vi "main.vi"() -> ()   [LabVIEW 2021]
uses:
  Global Config.ctl
  ini Entry.ctl
  VIPM.ctl
  <userlib>/_MGI/Application Control/MGI Gray if/MGI Gray if False.vi
  <vilib>/addons/_JKI.lib/Serialization/JSON/JKI JSON Serialization.lvlib
panel:
  out "Status":string
  out "Progress Bar":dbl(slide) scale=0.0..10.0
  in  "Start":bool
  in  "LV Install Folder":path caption="LabVIEW Installation Folder (eg: C:\\Program Files (x86)\\National Instruments\\LabVIEW 2021)"
  # "LV-Custom-Settings"
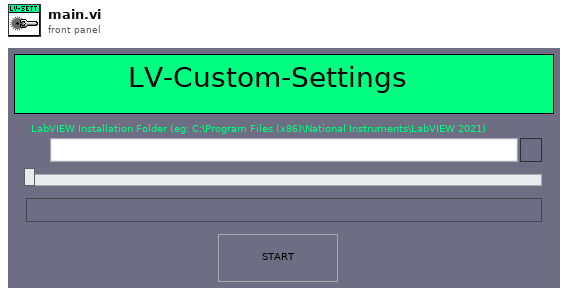
[diagram p1: front panel]
types:
  T1 = enum8{"Enabled", "Disabled", "Disabled and Grayed Out"}
  T2 = enum32{"Invalid", "Default", "Floating", "Floating/Auto-Hide", "Modal"}
  T3 = enum16{"open", "replace", "create", "open or create", "replace or create", "replace or create with confirmation"}
  T4 = typedef "Global Config.ctl" = cluster{"LabVIEW.ini":T5[], "VIPM":T6}
  T5 = typedef "ini Entry.ctl" = cluster{"section":string, "key":string, "value":variant}
  T6 = typedef "VIPM.ctl" = cluster{"official-packages":string[], "unofficial-package-urls":string[]}
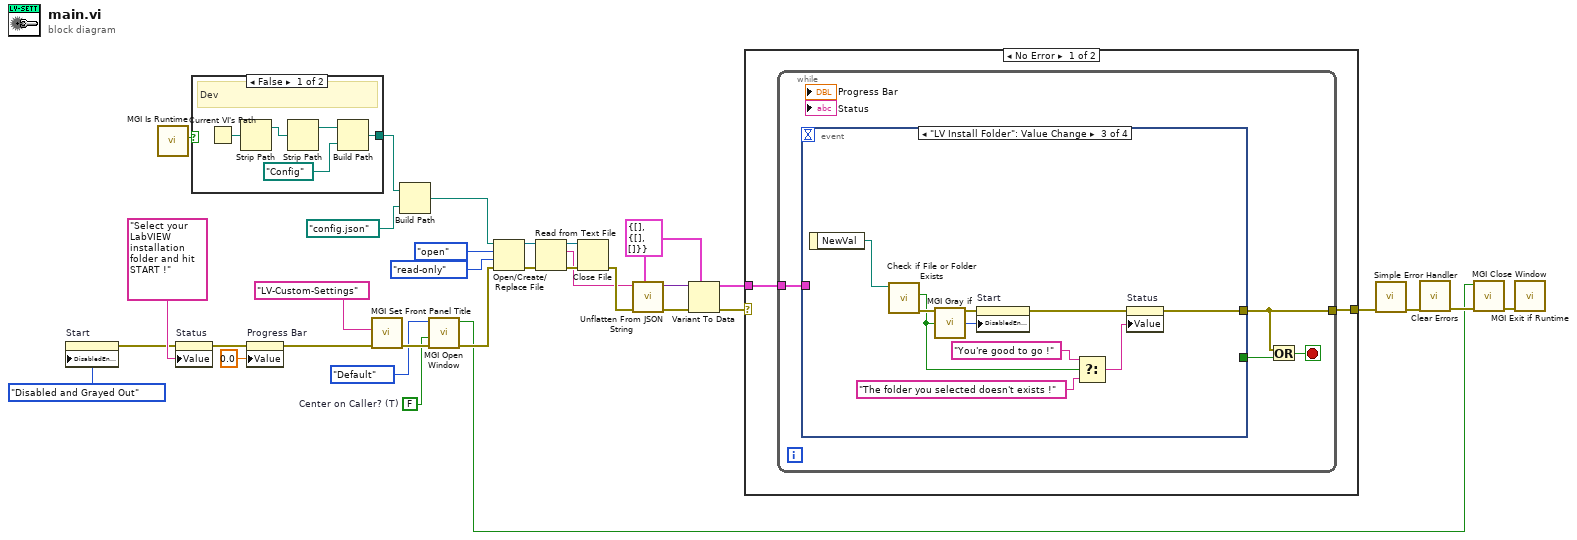
[diagram p0: block diagram]
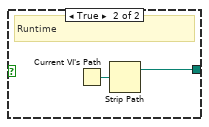
[diagram p2: hidden frame]
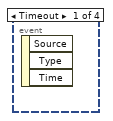
[diagram p3: hidden frame]
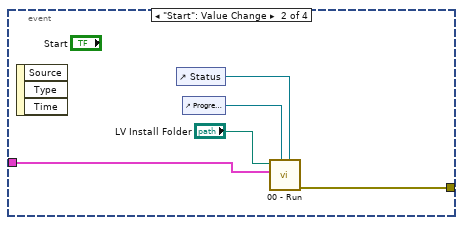
[diagram p4: hidden frame]
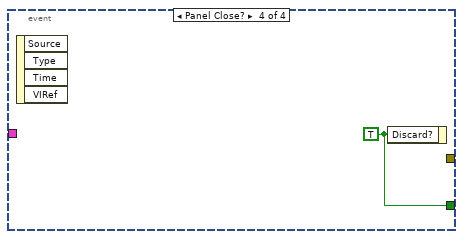
[diagram p5: hidden frame]
diagram:
  w7 = FALSE  # Center on Caller? (T)
  w20 = T4 {"LabVIEW.ini"=[], "VIPM"={"official-packages"=[], "unofficial-package-urls"=[]}} ("Global Config")
  n1 = property on="Start" class="Bool"("DisabledEnum"=T1."Disabled and Grayed Out" ("Disabled")) -> (error out=w5:errorcluster)  [unwired: 2 in, 1 out]
  n2 = call <userlib>:"MGI Is Runtime.vi"() -> ("Run Time System?"=w6:bool)  [unwired: 7 in]
  n3 = property on="Status" class="Str"(error in=w5, "Value"="Select your LabVIEW installation folder and hit START !" ("Status")) -> (error out=w15:errorcluster)  [unwired: 1 in, 1 out]
  n4 = case shown="False" w6 {
    tunnel: [w37 w39] -> w19
    frame False {
      # "Dev"
      n5 = Current VI's Path() -> (path=w38:path)
      n6 = Strip Path(path=w38) -> (stripped path=w35:path)  [unwired: 1 out]
      n7 = Strip Path(path=w35) -> (stripped path=w34:path)  [unwired: 1 out]
      n8 = Build Path(base path=w34, name or relative path=path "Config") -> (appended path=w37:path)
    }
    frame True {
      # "Runtime"
      n9 = Current VI's Path() -> (path=w40:path)
      n10 = Strip Path(path=w40) -> (stripped path=w39:path)  [unwired: 1 out]
    }
  }
  n11 = property on="Progress Bar" class="Slide (strict)"(error in=w15, "Value"=0.0 ("Progress Bar")) -> (error out=w2:errorcluster)  [unwired: 1 in, 1 out]
  n12 = call <userlib>:"MGI Set Front Panel Title.vi"("Error In"=w2, "Front Panel Window:Title"="LV-Custom-Settings") -> ("Error Out"=w10:errorcluster)  [unwired: 7 in, 1 out]
  n13 = Build Path(base path=w19, name or relative path=path "config.json") -> (appended path=w17:path)
  n14 = call <userlib>:"MGI Open Window.vi"("error in (no error)"=w10, "Center on Caller? (T)"=w7, "Behavior (Modal)"=T2."Default") -> ("error out"=w3:errorcluster, "Open Initially?"=w1:bool)  [unwired: 7 in]
  n15 = Open/Create/Replace File(file path (use dialog)=w17, error in=w3, operation (0:open)=T3."open", access (0:read/write)=enum16{"read/write", "read-only", "write-only"}."read-only") -> (refnum out=w30:refnum<file>, error out=w29:errorcluster)  [unwired: 2 in, 1 out]
  n16 = Read from Text File(file (use dialog)=w30, error in=w29) -> (refnum out=w28:refnum<file>, text=w23:string, error out=w27:errorcluster)  [unwired: 2 in, 1 out]
  n17 = Close File(refnum=w28, error in=w27) -> (error out=w26:errorcluster)  [unwired: 1 out]
  n18 = call <vilib>:"Unflatten From JSON String.vi"("Type and Defaults"=w20, "error in (no error)"=w26, "JSON String"=w23) -> ("error out"=w21:errorcluster, "Variant"=w22:variant)  [unwired: 7 in]
  n19 = Variant To Data(error in=w21, type=w20, Variant=w22) -> (data=w31:T4, error out=w32:errorcluster)
  n20 = case shown="No Error" w32 {
    selector: w32 -> [_ w62]
    tunnel: [w42 w62] -> w33
    tunnel: w31 -> [w41 _]
    frame No Error {
      n21 = while {
        tunnel: [w45] -> w42
        tunnel: w41 -> [w43]
        stop <- w46 stop-if-true
        n22 = event shown="[2] \"LV Install Folder\": Value Change" {
          selector: _ -> [_ _ _ _]
          dyn-events: _ -> [_ _ _ _]
          timeout: _ -> [_ _ _ _]
          tunnel: [_ w51 w56 _] -> w45
          tunnel: [_ _ _ w61] -> w44
          tunnel: w43 -> [_ w49 _ _]
          event Timeout {
            n23 = event-data() -> ()  [unwired: 1 in, 3 out]
          }
          event "Start": Value Change {
            n24 = event-data() -> ()  [unwired: 1 in, 3 out]
            n25 = control-ref of="Status"() -> (w47:refnum<vi>)
            n26 = control-ref of="Progress Bar"() -> (w48:refnum<vi>)
            n27 = call "00 - Run.vi"("Status Ref"=w47, "Progress Bar Ref"=w48, "Global Config"=w49, "LabVIEW Install Folder"="LV Install Folder") -> ("error out"=w51:errorcluster)  [unwired: 7 in]
          }
          event "LV Install Folder": Value Change {
            n28 = event-data() -> ("NewVal"=w60:path)  [unwired: 1 in]
            n29 = call <vilib>:"Check if File or Folder Exists.vi"("path"=w60) -> ("error out"=w59:errorcluster, "file or folder exists?"=w53:bool)  [unwired: 8 in, 1 out]
            n30 = call-poly <userlib>:"MGI Gray if.vi"("Boolean"=w53) -> ("Disabled"=w58:T1)
            n31 = property on="Start" class="Bool"(error in=w59, "DisabledEnum"=w58) -> (error out=w57:errorcluster)  [unwired: 1 in, 1 out]
            n32 = Select(t="You're good to go !", s=w53, f="The folder you selected doesn't exists !" ("Status")) -> (s? t:f=w55:string)
            n33 = property on="Status" class="Str"(error in=w57, "Value"=w55) -> (error out=w56:errorcluster)  [unwired: 1 in, 1 out]
          }
          event Panel Close? {
            w61 = TRUE ("Discard?")
            n34 = event-data() -> ()  [unwired: 1 in, 4 out]
            n35 = event-data("Discard?"=w61) -> ()  [unwired: 1 in, 1 out]
          }
        }
        n36 = Or(x=w45, y=w44) -> (x .or. y?=w46:bool)
      }
    }
    frame Error {
    }
  }
  n37 = call <vilib>:"Simple Error Handler.vi"("error in (no error)"=w33) -> ("error out"=w11:errorcluster)  [unwired: 4 in, 4 out]
  n38 = call <vilib>:"Clear Errors.vi"("error in (no error)"=w11) -> ("error out"=w13:errorcluster)  [unwired: 5 in, 1 out]
  n39 = call <userlib>:"MGI Close Window.vi"("error in (no error)"=w13, "Open Initially?"=w1) -> ("error out"=w12:errorcluster)  [unwired: 9 in]
  n40 = call <userlib>:"MGI Exit if Runtime.vi"("Error In (Dependency Only)"=w12) -> ()  [unwired: 11 in]
